vi "Configure Modulation (Digital).vi"(0 "VISA resource name":refnum<visa-resource-name>, 1 "Enable Digital Modulation (T:Enable)":bool=TRUE, 2 "Modulation Type (6: pi/4  DQPSK)":u16(ring)=6 items=["BPSK"=0, "QPSK"=1, "IS-95 QPSK"=2, "Gray Coded QPSK"=3, "OQPSK"=4, "IS-95 OQPSK"=5, "pi/4 DQPSK"=6, "8PSK"=7, "16PSK"=8, "D8PSK"=9, "MSK"=10, "2-Lvl FSK"=11, "4-Lvl FSK"=12, "8-Lvl FSK"=13, "16-Lvl FSK"=14, "C4FM"=15, "4QAM"=16, "16QAM"=17, "32QAM"=18, "64QAM"=19, "128QAM"=20, "256QAM"=21, "EDGE"=24], 3 "FSK Frequency Deviation (400 Hz)":dbl=400.0, 5 "Multicarrier Phase (0: Fixed)":u16(ring) items=["Fixed", "Random"], 7 "Standard (1: NADC)":u16(ring)=1 items=["GSM", "NADC", "PDC", "PHS", "DECT", "APCO 25 w/C4FM", "APCO w/CQPSK", "CDPD", "PWT", "EDGE", "TETRA", "Multicarrier", "Select File", "Bluetooth", "Default"], 9 "File Name (\"\")":string, 11 "error in (no error)":errorcluster, 12 "Symbol Rate (24.3 kbps)":dbl=24300.0, 13 "ASK Depth (100 percent)":dbl=100.0) -> (4 "VISA resource name out":refnum<visa-resource-name>, 15 "error out":errorcluster)   [LabVIEW 2011, in "Agilent PSG MXG Series.lvlib"]
doc: "Configures the state, modulation type, standard and symbol rate for the digital modulation.\n\n<B>Notes:</B>\n(1) This VI is valid only in E8267C, E8267D, N5182A.\n\n(2) For E8267C, this VI is valid only when the instrument installs <B>Option 002</B> (Internal baseband generator) or <B>Option 602</B> (Digital bus baseband generator).\n\n(3) For E8267D, this VI is valid only when the instrument installs <B>Option 601</B> or <B>Option 602</B> (Internal baseband generator).\n\n(4) For N5182A, this VI is valid only when the instrument installs <B>Option 651</B> or <B>Option 652</B> or <B>Option 654</B> (Internal baseband generator)."
uses:
  Agilent PSG MXG Series.lvlib
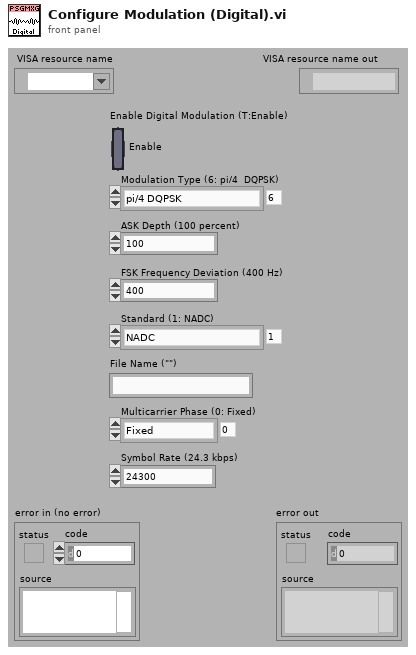
[diagram p1: front panel]
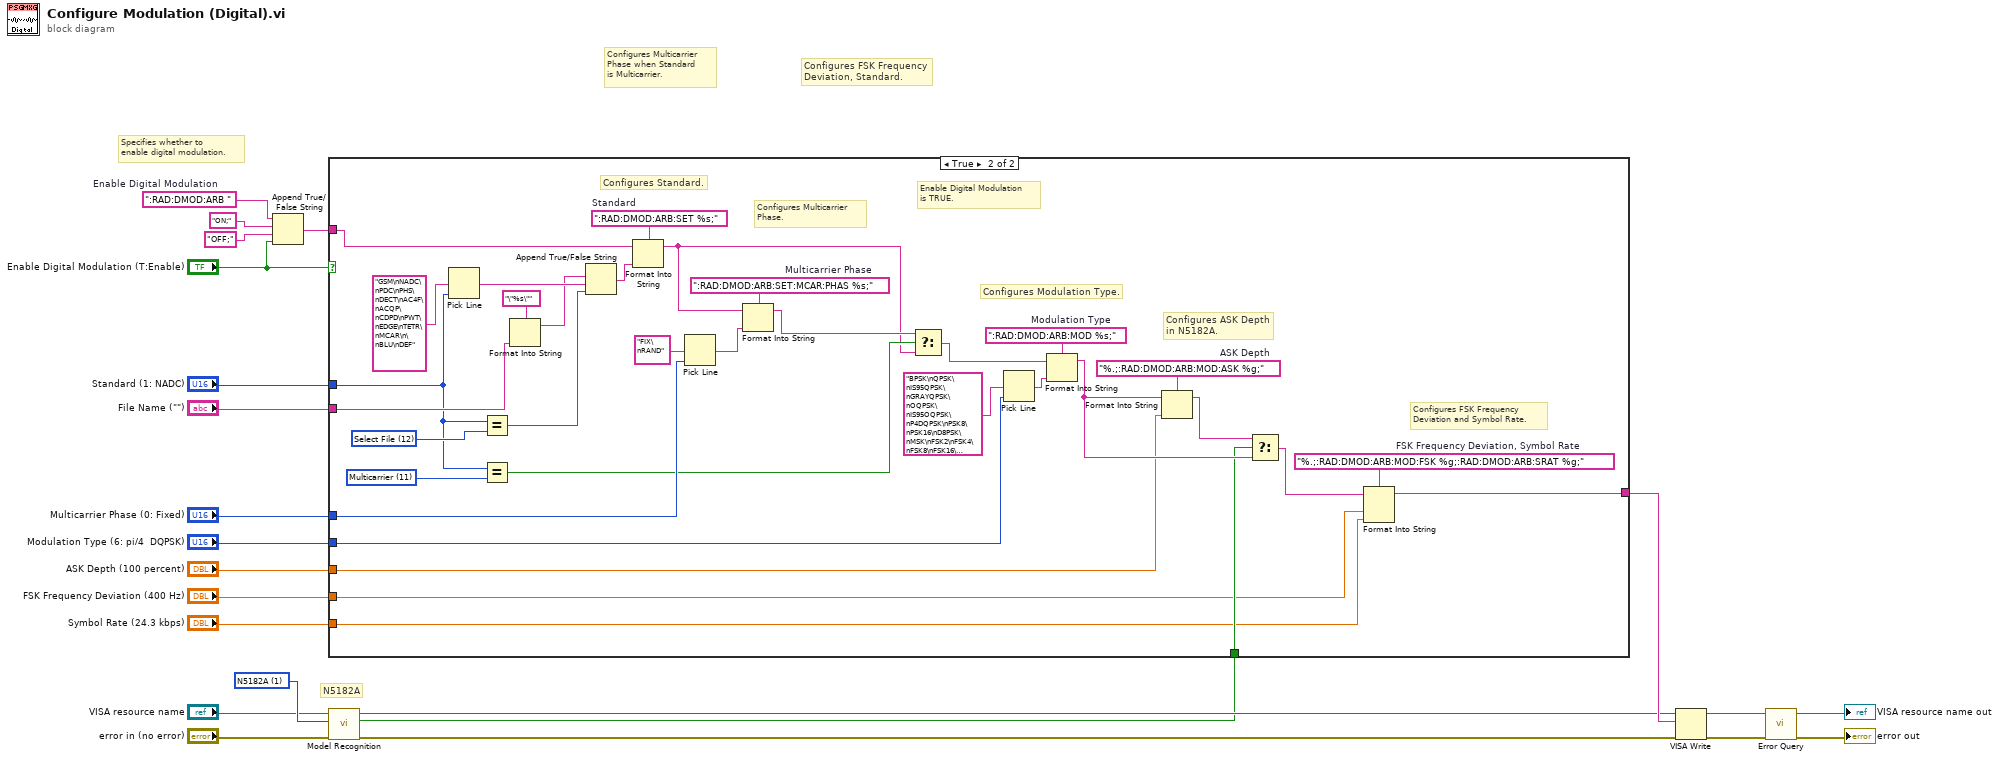
[diagram p0: block diagram]
diagram:
  w8 = u16 1 items=["N5181A"=0, "N5182A"=1, "E8241A"=5, "E8244A"=6, "E8251A"=7, "E8254A"=8, "E8247C"=10, "E8257C"=11, "E8267C"=12, "E8257D"=15, "E8267D"=16] ("Model Type (0: N5181A)")
  w23 = ":RAD:DMOD:ARB "  # Enable Digital Modulation
  # "Configures Multicarrier\nPhase when Standard\nis Multicarrier."
  # "Configures FSK Frequency\nDeviation, Standard."
  # "Specifies whether to\nenable digital modulation."
  # "N5182A"
  n1 = Append True/False String(1:"Enable Digital Modulation (T:Enable)", 2:"OFF;" ("false string"), 3:"ON;" ("true string"), 4:w23) -> (0:w19:string)
  n2 = call "Model Recognition.vi"("error in (no error)"="error in (no error)", "Model Type (0: N5181A)"=w8, "VISA resource name"="VISA resource name") -> ("error out"=w6:errorcluster, "Is Model Correct"=w5:bool, "VISA resource name out"=w7:refnum<visa-resource-name>)  [unwired: 6 in]
  n3 = case shown="True" "Enable Digital Modulation (T:Enable)" {
    tunnel: w19 -> [w24 w42]
    tunnel: "Modulation Type (6: pi/4  DQPSK)" -> [_ w28]
    tunnel: "FSK Frequency Deviation (400 Hz)" -> [_ w26]
    tunnel: "Standard (1: NADC)" -> [_ w47]
    tunnel: "File Name (\"\")" -> [_ w53]
    tunnel: "Multicarrier Phase (0: Fixed)" -> [_ w48]
    tunnel: "Symbol Rate (24.3 kbps)" -> [_ w25]
    tunnel: [w24 w43] -> w12
    tunnel: "ASK Depth (100 percent)" -> [_ w27]
    tunnel: w5 -> [_ w31]
    frame False {
      # "Enable Digital Modulation\nis FALSE."
    }
    frame True {
      w30 = "%.;:RAD:DMOD:ARB:MOD:FSK %g;:RAD:DMOD:ARB:SRAT %g;"  # FSK Frequency Deviation, Symbol Rate
      w36 = "%.;:RAD:DMOD:ARB:MOD:ASK %g;"  # ASK Depth
      w33 = ":RAD:DMOD:ARB:MOD %s;"  # Modulation Type
      w41 = ":RAD:DMOD:ARB:SET %s;"  # Standard
      w46 = u16 11 items=["GSM", "NADC", "PDC", "PHS", "DECT", "APCO 25 w/C4FM", "APCO w/CQPSK", "CDPD", "PWT", "EDGE", "TETRA", "Multicarrier", "Select File"] ("Setup (1: NADC)")
      w51 = ":RAD:DMOD:ARB:SET:MCAR:PHAS %s;"  # Multicarrier Phase
      w57 = u16 12 items=["GSM", "NADC", "PDC", "PHS", "DECT", "APCO 25 w/C4FM", "APCO w/CQPSK", "CDPD", "PWT", "EDGE", "TETRA", "Multicarrier", "Select File"] ("Setup (1: NADC)")
      # "Configures Multicarrier\nPhase."
      # "Configures Standard."
      # "Configures ASK Depth\nin N5182A."
      # "Configures Modulation Type."
      # "Configures FSK Frequency\nDeviation and Symbol Rate."
      # "Enable Digital Modulation\nis TRUE."
      n4 = Pick Line(multi-line string="GSM\nNADC\nPDC\nPHS\nDECT\nAC4F\nACQP\nCDPD\nPWT\nEDGE\nTETR\nMCAR\n\nBLU\nDEF", line index=w47) -> (output string=w55:string)  [unwired: 1 in]
      n5 = Equal?(x=w47, y=w57) -> (x = y?=w56:bool)
      n6 = Equal?(x=w47, y=w46) -> (x = y?=w44:bool)
      n7 = Format Into String(format string="\"%s\"", w53) -> (resulting string=w52:string)  [unwired: 2 in, 1 out]
      n8 = Append True/False String(1:w56, 2:w55, 3:w52) -> (0:w40:string)  [unwired: 1 in]
      n9 = Format Into String(format string=w41, initial string=w42, w40) -> (resulting string=w39:string)  [unwired: 1 in, 1 out]
      n10 = Pick Line(multi-line string="FIX\nRAND", line index=w48) -> (output string=w50:string)  [unwired: 1 in]
      n11 = Format Into String(format string=w51, initial string=w39, w50) -> (resulting string=w45:string)  [unwired: 1 in, 1 out]
      n12 = Select(t=w45, s=w44, f=w39) -> (s? t:f=w32:string)
      n13 = Pick Line(multi-line string="BPSK\nQPSK\nIS95QPSK\nGRAYQPSK\nOQPSK\nIS95OQPSK\nP4DQPSK\nPSK8\nPSK16\nD8PSK\nMSK\nFSK2\nFSK4\nFSK8\nFSK16\nC4FM\nQAM4\nQAM16\nQAM32\nQAM64\nQAM128\nQAM256\n\n\nEDGE", line index=w28) -> (output string=w34:string)  [unwired: 1 in]
      n14 = Format Into String(format string=w33, initial string=w32, w34) -> (resulting string=w38:string)  [unwired: 1 in, 1 out]
      n15 = Format Into String(format string=w36, initial string=w38, w27) -> (resulting string=w37:string)  [unwired: 1 in, 1 out]
      n16 = Select(t=w37, s=w31, f=w38) -> (s? t:f=w29:string)
      n17 = Format Into String(format string=w30, initial string=w29, w26, w25) -> (resulting string=w43:string)  [unwired: 1 in, 1 out]
    }
  }
  n18 = VISA Write(VISA resource name=w7, write buffer=w12, error in (no error)=w6) -> (VISA resource name out=w11:refnum<visa-resource-name>, error out=w10:errorcluster)  [unwired: 1 out]
  n19 = call "Error Query.vi"("error in (no error)"=w10, "VISA resource name"=w11) -> ("error out"=→"error out":errorcluster, "VISA resource name out"=→"VISA resource name out":refnum<visa-resource-name>)  [unwired: 6 in, 2 out]
